vi "Pololu-Slew Motor.vi"(1 "Servo Accel - Degreees/Sec^2":u16, 2 "Servo Speed - Degrees/Sec":u16, 4 "User Units-Max":u16=180, 5 "Servo Units-Max":u16=2416, 6 "User Units-Min":u16, 7 "Servo Units-Min":u16=576, 8 "error in":errorcluster, 9 "Servo Channel":u16, 10 "Position -User Units":u16(slide)=576 min=576 max=2416 scale=0.0..180.0, 11 "VISA resource name":refnum<visa-resource-name>) -> (0 "error out":errorcluster)   [LabVIEW 2018]
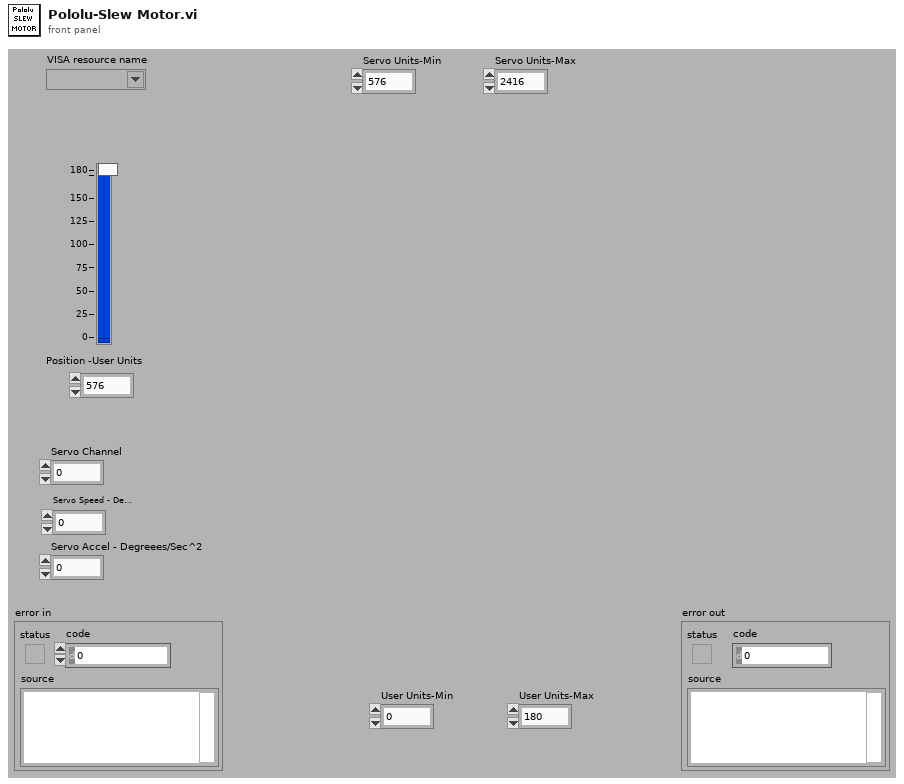
[diagram p1: front panel]
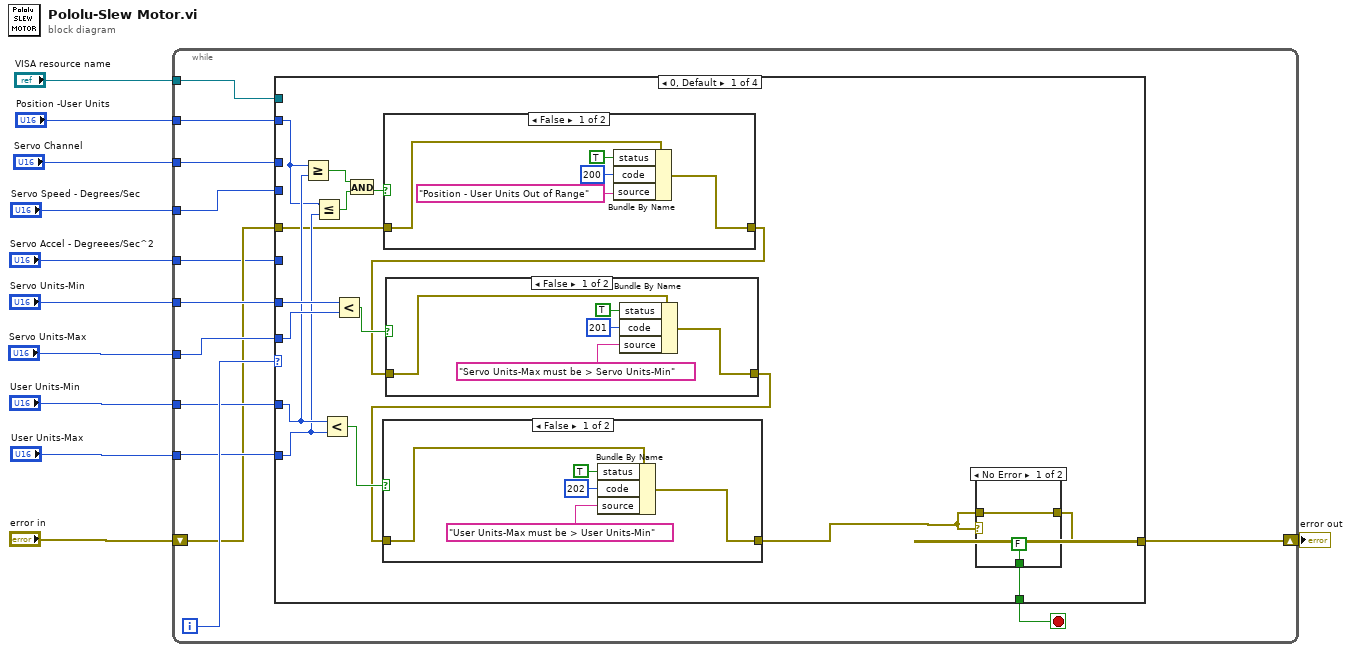
[diagram p0: block diagram]
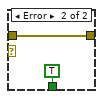
[diagram p2: hidden frame]
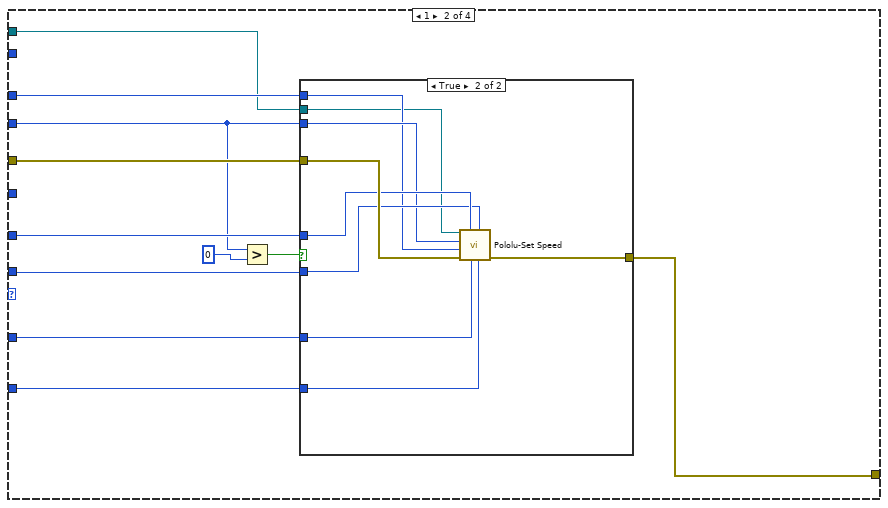
[diagram p6: hidden frame]
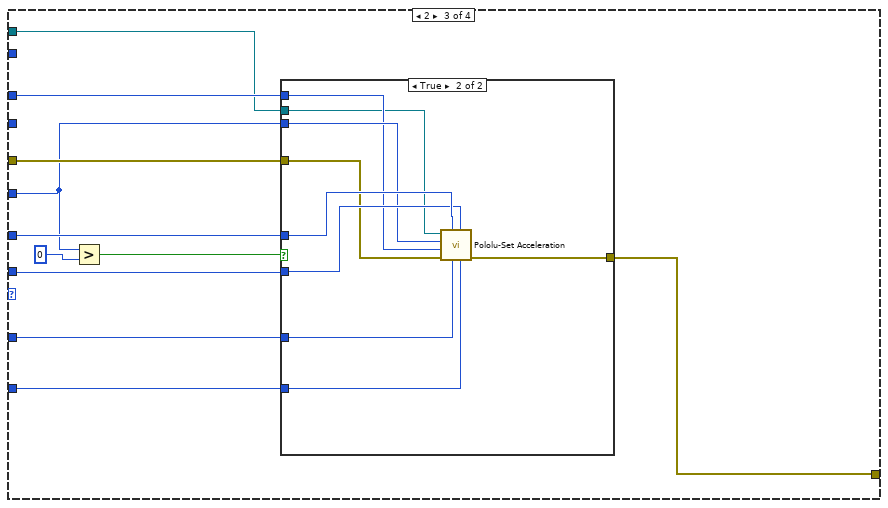
[diagram p8: hidden frame]
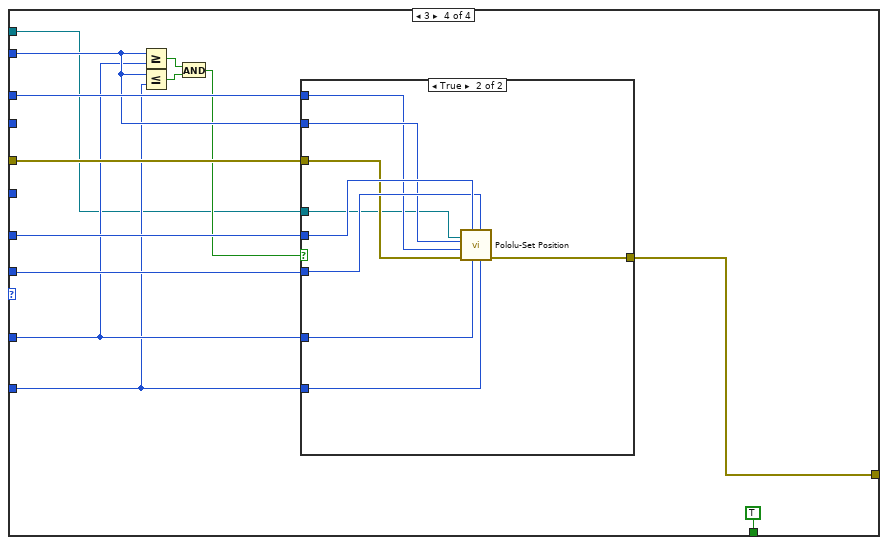
[diagram p10: hidden frame]
diagram:
  n1 = while {
    tunnel: "Position -User Units" -> [w23]
    tunnel: "Servo Units-Min" -> [w19]
    tunnel: "Servo Units-Max" -> [w22]
    tunnel: "User Units-Min" -> [w21]
    tunnel: "User Units-Max" -> [w20]
    shift-right: [w16] -> w5
    shift-left: "error in" -> [w18]
    tunnel: "Servo Speed - Degrees/Sec" -> [w13]
    tunnel: "Servo Channel" -> [w15]
    tunnel: "Servo Accel - Degreees/Sec^2" -> [w14]
    tunnel: "VISA resource name" -> [w12]
    i -> [w24]
    stop <- w17 stop-if-true
    n2 = case shown="0, Default" w24 {
      tunnel: w23 -> [w37 _ _ w111]
      tunnel: w19 -> [w40 w71 w92 w115]
      tunnel: w22 -> [w39 w70 w91 w114]
      tunnel: w21 -> [w38 w69 w90 w107]
      tunnel: w20 -> [w36 w68 w89 w106]
      tunnel: w18 -> [w30 w72 w93 w116]
      tunnel: [w27 _ _ TRUE] -> w17
      tunnel: [w26 w67 w88 w113] -> w16
      tunnel: w13 -> [_ w66 _ _]
      tunnel: w15 -> [_ w73 w94 w117]
      tunnel: w14 -> [_ _ w85 _]
      tunnel: w12 -> [_ w63 w84 w105]
      frame 0, Default {
        n3 = Greater Or Equal?(x=w37, y=w38) -> (x >= y?=w34:bool)
        n4 = Less Or Equal?(x=w37, y=w36) -> (x <= y?=w35:bool)
        n5 = Less?(x=w38, y=w36) -> (x < y?=w31:bool)
        n6 = Less?(x=w40, y=w39) -> (x < y?=w32:bool)
        n7 = And(x=w34, y=w35) -> (x .and. y?=w33:bool)
        n8 = case shown="False" w33 {
          tunnel: w30 -> [w49 w50]
          tunnel: [w45 w50] -> w29
          frame False {
            n9 = Bundle By Name(cluster=w49, "status"=TRUE, "code"=200, "source"="Position - User Units Out of Range") -> (w45:errorcluster)
          }
          frame True {
          }
        }
        n10 = case shown="False" w32 {
          tunnel: w29 -> [w52 w56]
          tunnel: [w51 w56] -> w28
          frame False {
            n11 = Bundle By Name(cluster=w52, "status"=TRUE, "code"=201, "source"="Servo Units-Max must be > Servo Units-Min") -> (w51:errorcluster)
          }
          frame True {
          }
        }
        n12 = case shown="False" w31 {
          tunnel: w28 -> [w58 w62]
          tunnel: [w57 w62] -> w25
          frame False {
            n13 = Bundle By Name(cluster=w58, "status"=TRUE, "code"=202, "source"="User Units-Max must be > User Units-Min") -> (w57:errorcluster)
          }
          frame True {
          }
        }
        n14 = case shown="No Error" w25 {
          tunnel: [FALSE TRUE] -> w27
          tunnel: w25 -> [w42 w43]
          tunnel: [w42 w43] -> w26
          frame No Error {
          }
          frame Error {
          }
        }
      }
      frame 1 {
        n15 = Greater?(x=w66, y=u16 0) -> (0:w64:bool)
        n16 = case shown="True" w64 {
          tunnel: w66 -> [_ w77]
          tunnel: w73 -> [_ w76]
          tunnel: w72 -> [w74 w83]
          tunnel: w71 -> [_ w82]
          tunnel: w70 -> [_ w81]
          tunnel: w69 -> [_ w80]
          tunnel: w68 -> [_ w79]
          tunnel: [w74 w78] -> w67
          tunnel: w63 -> [_ w75]
          frame False {
          }
          frame True {
            n17 = call "Pololu-Set Speed.vi"("User Scale Max"=w79, "Servo Units Max"=w81, "User Scale Min"=w80, "Servo Units Min"=w82, "error in"=w83, "Servo Chan"=w76, "Velocity (deg/sec)"=w77, "VISA resource name"=w75) -> ("error out"=w78:errorcluster)  [unwired: 3 in]
          }
        }
      }
      frame 2 {
        n18 = Greater?(x=w85, y=u16 0) -> (0:w86:bool)
        n19 = case shown="True" w86 {
          tunnel: w85 -> [_ w98]
          tunnel: w94 -> [_ w97]
          tunnel: w93 -> [w95 w101]
          tunnel: w92 -> [_ w104]
          tunnel: w91 -> [_ w103]
          tunnel: w90 -> [_ w102]
          tunnel: w89 -> [_ w99]
          tunnel: [w95 w100] -> w88
          tunnel: w84 -> [_ w96]
          frame False {
          }
          frame True {
            n20 = call "Pololu-Set Acceleration.vi"("User Units Max"=w99, "Servo Units Max"=w103, "User Units Min"=w102, "Servo Units Min"=w104, "error in"=w101, "Servo Chan"=w97, "Acceleration (deg/sec^2)"=w98, "VISA resource name"=w96) -> ("error out"=w100:errorcluster)  [unwired: 3 in]
          }
        }
      }
      frame 3 {
        n21 = Greater Or Equal?(x=w111, y=w107) -> (x >= y?=w109:bool)
        n22 = Less Or Equal?(x=w111, y=w106) -> (x <= y?=w110:bool)
        n23 = And(x=w109, y=w110) -> (x .and. y?=w108:bool)
        n24 = case shown="True" w108 {
          tunnel: w111 -> [_ w121]
          tunnel: w117 -> [_ w120]
          tunnel: w116 -> [w118 w124]
          tunnel: w115 -> [_ w127]
          tunnel: w114 -> [_ w126]
          tunnel: w107 -> [_ w125]
          tunnel: w106 -> [_ w122]
          tunnel: [w118 w123] -> w113
          tunnel: w105 -> [_ w119]
          frame False {
          }
          frame True {
            n25 = call "Pololu-Set Position.vi"("User Units Max"=w122, "Servo Units Max"=w126, "User Units Min"=w125, "Servo Units Min"=w127, "error in"=w124, "Servo Chan"=w120, "position"=w121, "VISA resource name"=w119) -> ("error out"=w123:errorcluster)  [unwired: 3 in]
          }
        }
      }
    }
  }
  "error out" <- w5
